vi "auto_hold.vi"(8 "averages":i32=50 min=1, 9 "trigger rate (Hz)":dbl=25.0, 10 "hold_off":u32=2000 caption="hold off (in)", 11 "auto_hold":bool=TRUE caption="super_shuffle?") -> (2 "hold_off (out)":u32=2000 caption="hold off (out)")   [LabVIEW 2017, in "tools.lvlib"]
uses:
  tools.lvlib
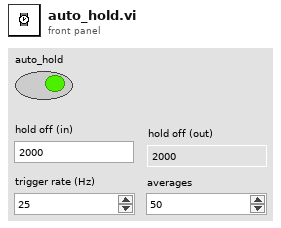
[diagram p1: front panel]
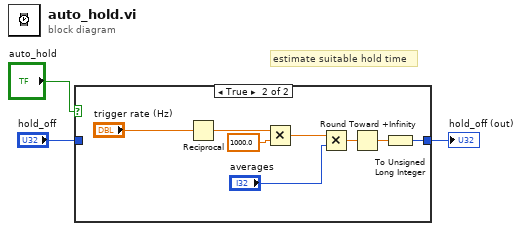
[diagram p0: block diagram]
diagram:
  # "estimate suitable hold time"
  n1 = case shown="True" "auto_hold" {
    tunnel: "hold_off" -> [w4 _]
    tunnel: [w4 w6] -> w2
    frame False {
    }
    frame True {
      n2 = Reciprocal(x="trigger rate (Hz)") -> (1/x=w12:dbl)
      n3 = Multiply(x=w12, y=1000.0) -> (x*y=w10:dbl)
      n4 = Multiply(x=w10, y="averages") -> (x*y=w9:dbl)
      n5 = Round Toward +Infinity(x=w9) -> (ceil(x): smallest int >= x=w8:dbl)
      n6 = To Unsigned Long Integer(number=w8) -> (unsigned 32bit integer=w6:u32)
    }
  }
  "hold_off (out)" <- w2
